vi "Remote Restart Cameras.vi"() -> (0 "Error out":errorcluster)   [LabVIEW 2015]
uses:
  Globals/CamServer global.vi
panel:
  # "PN 20/04/16"
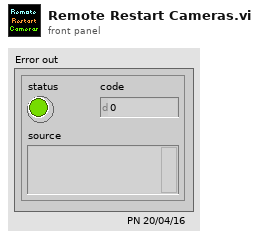
[diagram p1: front panel]
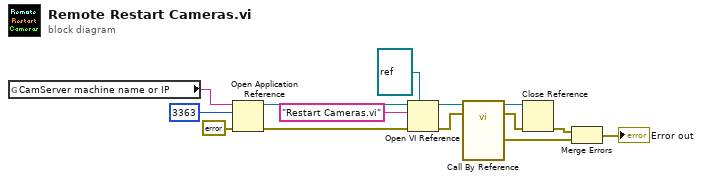
[diagram p0: block diagram]
diagram:
  n1 = global read "CamServer global.vi" "CamServer machine name or IP"() -> (w2:string)
  n2 = Open Application Reference(8:errorcluster {"status"=FALSE, "code"=0, "source"=""} ("error in (no error)"), 10:u16 3363 ("port"), 11:w2) -> (0:w1:errorcluster, 3:w12:refnum<vi>)  [unwired: 1 in]
  n3 = Open VI Reference(type specifier VI Refnum (for type only)=refnum<vi> refnum, application reference (local)=w12, vi path="Restart Cameras.vi" ("machine name"), error in (no error)=w1) -> (vi reference=w10:refnum<vi>, error out=w11:errorcluster)  [unwired: 2 in]
  n4 = call-by-ref "?"(reference=w10, error in=w11) -> (reference out=w9:refnum<vi>, error out=w8:errorcluster, "Error Out"=w7:errorcluster)
  n5 = Close Reference(reference=w9, error in (no error)=w8) -> (error out=w6:errorcluster)
  n6 = Merge Errors(w6, w7) -> (→"Error out":errorcluster)
